vi "SetDeviceAddress.vi"(8 "error in (no error)":errorcluster, 9 "Device Address":i32, 10 "DeviceKey In":string, 11 "CmdLib In":refnum<k24>) -> (0 "error out":errorcluster, 1 "New Device Address":i32, 2 "DeviceKey Out":string, 3 "CmdLib Out":refnum<k24>)   [LabVIEW 2019]
uses:
  C:/Users/jyxks/OneDrive/Documents/Program Files/New Focus/New Focus Picomotor Application/Samples/LabVIEW/Model 8742/LabVIEW 2009/CmdLib.dll
  Program Files/New Focus/New Focus Picomotor Application/Samples/LabVIEW/Model 8742/LabVIEW 2009/CmdLib.dll
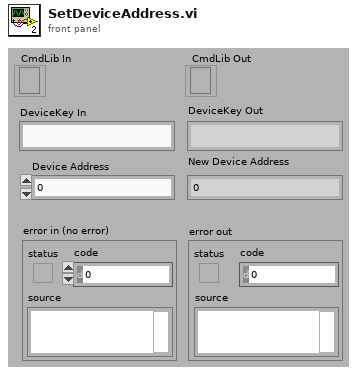
[diagram p1: front panel]
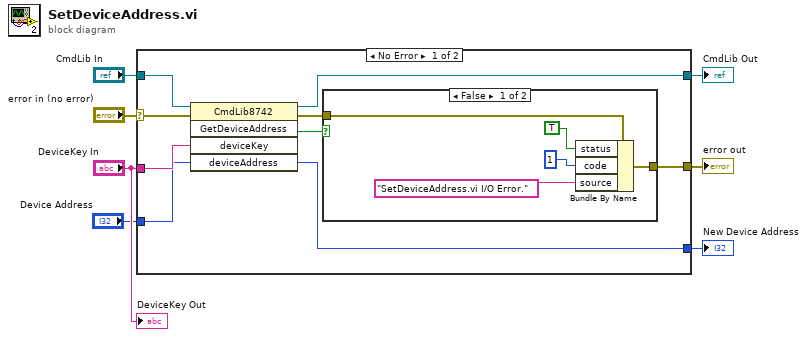
[diagram p0: block diagram]
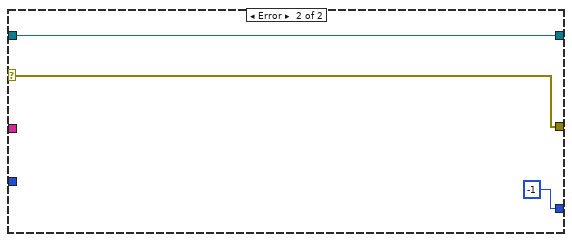
[diagram p3: hidden frame]
diagram:
  n1 = case shown="No Error" "error in (no error)" {
    selector: "error in (no error)" -> [w13 w24]
    tunnel: "CmdLib In" -> [w16 w25]
    tunnel: [w15 w25] -> w6
    tunnel: "DeviceKey In" -> [w14 _]
    tunnel: [w10 w24] -> w3
    tunnel: [w9 -1] -> w2
    tunnel: "Device Address" -> [w8 _]
    frame No Error {
      n2 = invoke class="CmdLib8742" method="GetDeviceAddress"(reference=w16, error in=w13, "deviceKey"=w14, "deviceAddress"=w8) -> (reference out=w15:refnum<k24>, error out=w11:errorcluster, "GetDeviceAddress"=w12:bool, "deviceAddress"=w9:i32)  [unwired: 1 in, 1 out]
      n3 = case shown="False" w12 {
        tunnel: w11 -> [w21 w22]
        tunnel: [w20 w22] -> w10
        frame False {
          n4 = Bundle By Name(cluster=w21, "status"=TRUE, "code"=1, "source"="SetDeviceAddress.vi I/O Error.") -> (w20:errorcluster)
        }
        frame True {
        }
      }
    }
    frame Error {
    }
  }
  "error out" <- w3
  "CmdLib Out" <- w6
  "New Device Address" <- w2
  "DeviceKey Out" <- "DeviceKey In"
